vi "Get_TCR.vi"(8 "error in":errorcluster, 11 "VISA name":refnum<visa-resource-name>) -> (0 "error out":errorcluster, 1 "valid":bool, 2 "TCR /ppm":dbl, 3 "VISA out":refnum<visa-resource-name>)   [LabVIEW 2018, in "QR-10x.lvlib"]
uses:
  QR-10x.lvlib
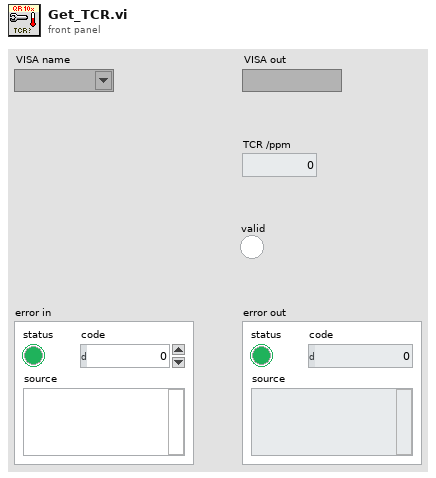
[diagram p1: front panel]
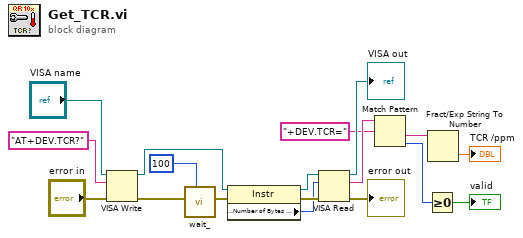
[diagram p0: block diagram]
diagram:
  n1 = VISA Write(VISA resource name="VISA name", write buffer="AT+DEV.TCR?", error in (no error)="error in") -> (VISA resource name out=w15:refnum<visa-resource-name>, error out=w9:errorcluster)  [unwired: 1 out]
  n2 = call "wait_.vi"("milliseconds to wait"=u32 100, "error in"=w9) -> ("error out"=w8:errorcluster)  [unwired: 9 in]
  n3 = property class="Instr"(reference=w15, error in=w8) -> (reference out=w11:refnum<visa-resource-name>, error out=w13:errorcluster, "Serial Settings:Number of Bytes at Serial Port"=w12:u32)
  n4 = VISA Read(VISA resource name=w11, byte count=w12, error in (no error)=w13) -> (VISA resource name out=→"VISA out":refnum<visa-resource-name>, read buffer=w6:string, error out=→"error out":errorcluster)  [unwired: 1 out]
  n5 = Match Pattern(string=w6, regular expression="+DEV.TCR=") -> (after substring=w4:string, offset past match=w3:i32)  [unwired: 1 in, 2 out]
  n6 = Greater Or Equal To 0?(x=w3) -> (x >= 0?=→"valid":bool)
  n7 = Fract/Exp String To Number(string=w4) -> (number=→"TCR /ppm":dbl)  [unwired: 3 in, 1 out]
